vi "derivativeFilter.vi"(10 "eta":dbl[](array[numeric])) -> (0 "nu_dot_hat":dbl[](array[numeric]), 3 "nu_hat":dbl[](array[numeric]))   [LabVIEW 2014]
uses:
  <vilib>/imath/engines/lvmath2/RunTimeEngine/ArithmeticOperatorToken/NIMS_ArithmeticOperator_minus.vi
  <instcachedir>/0/NIMS_ArithmeticOperator_minus_39C0593E74DA4138ACA2AB742906488D.lvgen/NIMS_ArithmeticOperator_minus_39C0593E74DA4138ACA2AB742906488D_003.vi
  <vilib>/imathl/engines/lvmath/Functions/Error Handling/Create Error.vi
  <vilib>/imath/engines/lvmath2/RunTimeEngine/NodeEndStatement/NIMS_NodeEndStatement_Output.vi
  <instcachedir>/0/NIMS_NodeEndStatement_Output_53EC0D466D134D7ABD903AC30B43404B.lvgen/NIMS_NodeEndStatement_Output_53EC0D466D134D7ABD903AC30B43404B_005.vi
  <vilib>/imath/engines/lvmath2/RunTimeEngine/ErrorHandling/NIMS_Finalize Error.vi
  <vilib>/imath/engines/lvmath2/RunTimeEngine/ArithmeticOperatorToken/NIMS_ArithmeticOperator_multmx(M,CV).vi
  <instcachedir>/0/NIMS_ArithmeticOperator_multmx(M,CV)_787B4652E60B4C52835A7FB23671E425.lvgen/NIMS_ArithmeticOperator_multmx(M,CV)_787B4652E60B4C52835A7FB23671E425_000.vi
  <instcachedir>/0/NIMS_NodeEndStatement_Output_53EC0D466D134D7ABD903AC30B43404B.lvgen/NIMS_NodeEndStatement_Output_53EC0D466D134D7ABD903AC30B43404B_002.vi
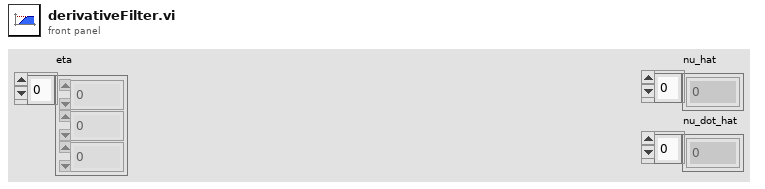
[diagram p1: front panel]
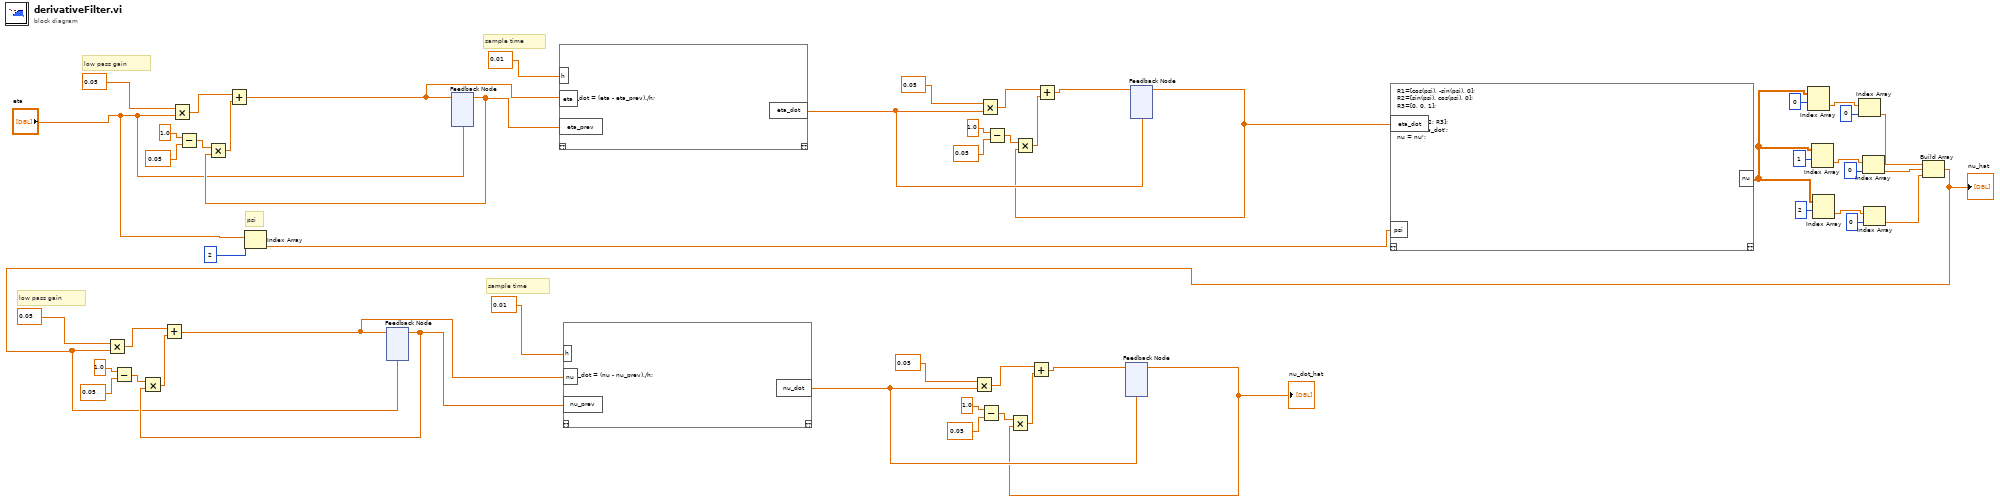
[diagram p0: block diagram]
diagram:
  # "low pass gain"
  # "sample time"
  # "psi"
  # "low pass gain"
  # "sample time"
  n1 = Subtract(x=1.0, y=0.05) -> (x-y=w15:dbl)
  n2 = Multiply(x=0.05, y="eta") -> (x*y=w53:dbl[])
  n3 = Subtract(x=1.0, y=0.05) -> (x-y=w48:dbl)
  n4 = Index Array(array="eta", index=2) -> (element=w34:dbl)
  n5 = feedback #1("eta") -> (w46:dbl[])
  n6 = Multiply(x=w48, y=w46) -> (x*y=w50:dbl[])
  n7 = Add(x=w53, y=w50) -> (x+y=w45:dbl[])
  n8 = feedback-in #1(w45) -> ()
  n9 = mathscript code="eta_dot = (eta - eta_prev)./h;"("h"=0.01, "eta"=w45, "eta_prev"=w46) -> ("eta_dot"=w38:dbl[])  [unwired: 1 in, 1 out]
  n10 = Multiply(x=0.05, y=w38) -> (x*y=w44:dbl[])
  n11 = Subtract(x=1.0 ("Constant 2"), y=0.05 ("Constant 3")) -> (x-y=w6:dbl)
  n12 = Subtract(x=1.0 ("Constant 2"), y=0.05 ("Constant 3")) -> (x-y=w40:dbl)
  n13 = feedback #2(w38) -> (w2:dbl[])
  n14 = Multiply ("Multiply 2")(x=w40, y=w2) -> (x*y=w42:dbl[])
  n15 = Add(x=w44, y=w42) -> (x+y=w37:dbl[])
  n16 = feedback-in #2(w37) -> ()
  n17 = mathscript code="R1=[cos(psi), -sin(psi), 0];\nR2=[sin(psi), cos(psi), 0];\nR3=[0, 0, 1];\n\nR = [R1; R2; R3];\nnu = R*eta_dot';\nnu = nu';"("eta_dot"=w2, "psi"=w34) -> ("nu"=w24:dbl[][])  [unwired: 1 in, 1 out]
  n18 = Index Array(array=w24, index (row)=0) -> (element=w31:dbl[])  [unwired: 1 in]
  n19 = Index Array(array=w24, index (row)=1) -> (element=w28:dbl[])  [unwired: 1 in]
  n20 = Index Array(array=w24, index (row)=2) -> (element=w25:dbl[])  [unwired: 1 in]
  n21 = Index Array(array=w31, index=0) -> (element=w23:dbl)
  n22 = Index Array(array=w28, index=0) -> (element=w22:dbl)
  n23 = Index Array(array=w25, index=0) -> (element=w21:dbl)
  n24 = Build Array(w23, w22, w21) -> (w11:dbl[])
  "nu_hat" <- w11
  n25 = Multiply(x=0.05, y=w11) -> (x*y=w20:dbl[])
  n26 = feedback #3(w11) -> (w12:dbl[])
  n27 = Multiply(x=w15, y=w12) -> (x*y=w17:dbl[])
  n28 = Add(x=w20, y=w17) -> (x+y=w13:dbl[])
  n29 = feedback-in #3(w13) -> ()
  n30 = mathscript code="nu_dot = (nu - nu_prev)./h;"("h"=0.01, "nu"=w13, "nu_prev"=w12) -> ("nu_dot"=w3:dbl[])  [unwired: 1 in, 1 out]
  n31 = Multiply(x=0.05, y=w3) -> (x*y=w10:dbl[])
  n32 = feedback #4(w3) -> (w1:dbl[])
  "nu_dot_hat" <- w1
  n33 = Multiply ("Multiply 2")(x=w6, y=w1) -> (x*y=w8:dbl[])
  n34 = Add(x=w10, y=w8) -> (x+y=w4:dbl[])
  n35 = feedback-in #4(w4) -> ()
